vi "test malleable float to bytes v2.vi"() -> ()   [LabVIEW 2018, in "LV-Julia_ZMQ-Roundtrip_lib.lvlib"]
uses:
  LV-Julia_ZMQ-Roundtrip_lib.lvlib
  Bindata description.ctl
  64f9d793-bb93-41fe-8723-108ede85f934.vi
  0fbc5065-3fc2-4b1a-ac98-8b0d647fb522.vi
  64f9d793-bb93-41fe-8723-108ede85f934.vi/9d313e8a-9224-457f-a906-4ab8a5a19c99.vi
  0fbc5065-3fc2-4b1a-ac98-8b0d647fb522.vi/91456061-b3d7-4feb-9ee0-ac716754e4c9.vi
  check ID validity.vi
panel:
  out "bindata 1":u8[](array[numeric])
  out "bindata 2":u8[](array[numeric])
  out "flattened array 2":dbl[](array[numeric])
  in  "Tag 2":string="tg2"
  in  "Array 2":u32[](array[numeric])
  out "Bindata & descr out":cluster{"bindata_descr":T1[], "bindata":u8[]}
  out "error out":errorcluster
  in  "Tag 1":string="tg1"
  out "flattened array 1":dbl[](array[numeric])
  in  "Array 1":sgl[](array[numeric])
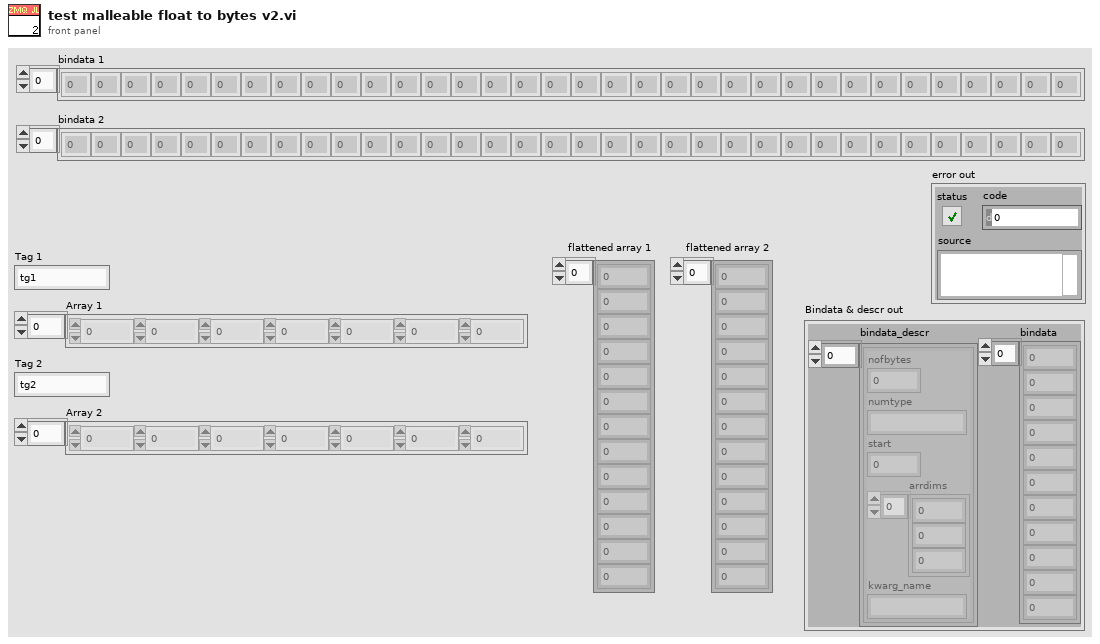
[diagram p1: front panel]
types:
  T1 = typedef "LV-Julia_ZMQ-Roundtrip_lib.lvlib/Bindata description.ctl" = cluster{"nofbytes":i32, "numtype":string, "start":i32, "arrdims":i32[], "kwarg_name":string}
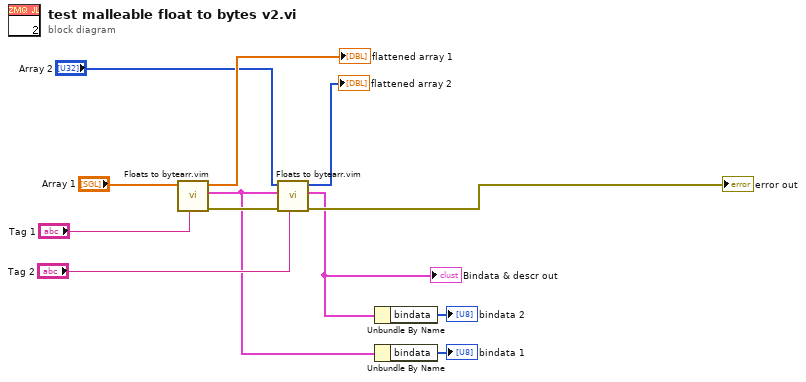
[diagram p0: block diagram]
diagram:
  n1 = call "Floats to bytearr.vim"("Tag"="Tag 1", "Array in"="Array 1") -> ("error out"=w9:errorcluster, "Bindata & descr out"=w1:cluster{"bindata_descr":T1[], "bindata":u8[]}, "flattened array out"=→"flattened array 1":sgl[])  [unwired: 7 in]
  n2 = call "Floats to bytearr.vim"("Tag"="Tag 2", "error in (no error)"=w9, "Bindata & descr in"=w1, "Array in"="Array 2") -> ("error out"=→"error out":errorcluster, "Bindata & descr out"=w4:cluster{"bindata_descr":T1[], "bindata":u8[]}, "flattened array out"=→"flattened array 2":u32[])  [unwired: 5 in]
  "Bindata & descr out" <- w4
  n3 = Unbundle By Name(w4) -> ("bindata"=→"bindata 2":u8[])
  n4 = Unbundle By Name(w1) -> ("bindata"=→"bindata 1":u8[])
